vi "SetColorStrToStrCtrl2.vi"(0 "ref string":refnum<vi>, 1 "string":string, 2 "result":string) -> ()   [LabVIEW 2018, in "Library-Ctrl.lvlib"]
uses:
  Library-Ctrl.lvlib
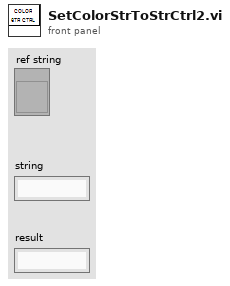
[diagram p1: front panel]
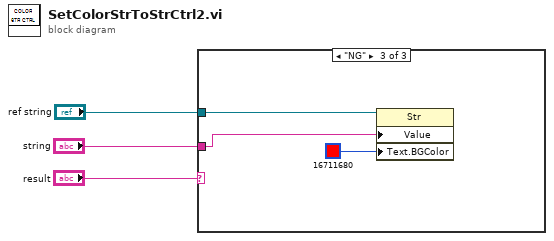
[diagram p0: block diagram]
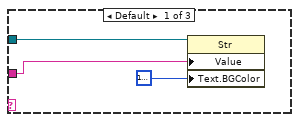
[diagram p2: hidden frame]
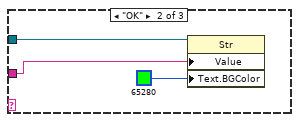
[diagram p3: hidden frame]
diagram:
  n1 = case shown="\"NG\"" "result" {
    tunnel: "ref string" -> [w6 w9 w12]
    tunnel: "string" -> [w4 w7 w10]
    frame Default {
      n2 = property class="Str"(reference=w6, "Value"=w4, "Text.BGColor"=u32 16777225) -> ()  [unwired: 1 in, 2 out]
    }
    frame "OK" {
      n3 = property class="Str"(reference=w9, "Value"=w7, "Text.BGColor"=u32 65280) -> ()  [unwired: 1 in, 2 out]
    }
    frame "NG" {
      n4 = property class="Str"(reference=w12, "Value"=w10, "Text.BGColor"=u32 16711680) -> ()  [unwired: 1 in, 2 out]
    }
  }
